vi "RSZVB Set Limit Check.vi"(7 "Limit Check (F: Off)":bool, 8 "error in (no error)":errorcluster {"code" format="%.0x"}, 9 "Limit Line (3: All)":i32(ring)=3 items=["Upper"=1, "Lower"=2, "All"=3], 10 "Channel (Trace) (1)":i32=1, 11 "VISA session":refnum<visa-resource-name>) -> (0 "error out":errorcluster {"code" format="%.0x"}, 3 "dup VISA session":refnum<visa-resource-name>)   [LabVIEW 2011]
doc: "This VI switches the limit check (or individual upper and lower limits) on or off.\n\nRemote-control command(s):\nCALCulate<Ch/Tr>:LIMit:STATe <Boolean>\nCALCulate<Ch/Tr>:LIMit:LOWer:STATe <Boolean>\nCALCulate<Ch/Tr>:LIMit:UPPer:STATe <Boolean>"
panel:
  # "On\nOff"
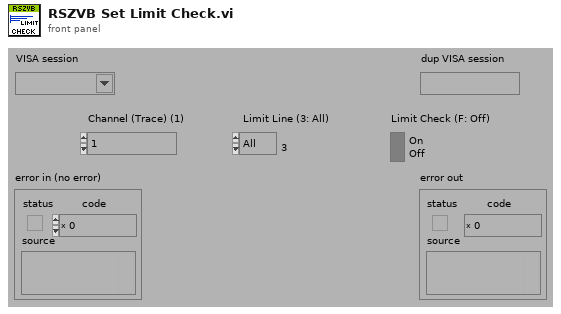
[diagram p1: front panel]
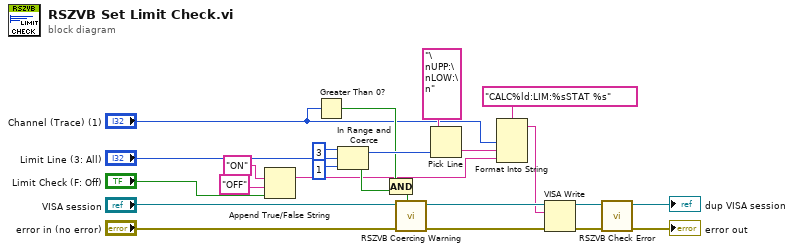
[diagram p0: block diagram]
diagram:
  n1 = Append True/False String(1:"Limit Check (F: Off)", 2:"OFF", 3:"ON") -> (0:w1:string)  [unwired: 1 in]
  n2 = Greater Than 0?(x="Channel (Trace) (1)") -> (x > 0?=w13:bool)
  n3 = In Range and Coerce(upper limit=3, x="Limit Line (3: All)", lower limit=1) -> (coerced(x)=w21:i32, In Range?=w14:bool)
  n4 = Compound Arithmetic op=AND(w13, w14) -> (w12:bool)
  n5 = call "RSZVB Coercing Warning.vi"("In Range?"=w12, "error in (no error)"="error in (no error)", "VISA session"="VISA session") -> ("error out"=w18:errorcluster, "dup VISA session"=w19:refnum<visa-resource-name>)  [unwired: 7 in]
  n6 = Pick Line(multi-line string="\nUPP:\nLOW:\n", line index=w21) -> (output string=w15:string)  [unwired: 1 in]
  n7 = Format Into String(format string="CALC%ld:LIM:%sSTAT %s", "Channel (Trace) (1)", w15, w1) -> (resulting string=w11:string)  [unwired: 2 in, 1 out]
  n8 = VISA Write(VISA resource name=w19, write buffer=w11, error in (no error)=w18) -> (VISA resource name out=w16:refnum<visa-resource-name>, error out=w17:errorcluster)  [unwired: 1 out]
  n9 = call "RSZVB Check Error.vi"("error in (no error)"=w17, "VISA session"=w16) -> ("error out"=→"error out":errorcluster, "dup VISA session"=→"dup VISA session":refnum<visa-resource-name>)  [unwired: 8 in]
